vi "Initialize.vi"(8 "error in (no error)":errorcluster, 11 "Configuration":T1) -> (0 "error out":errorcluster, 3 "Configuration Out":T1={"Data Tree Ref"=refnum, "FP Ref"=refnum, "Column Data Type"=[], "Search Clones Up To"=100, "SortOptions"={"Col.pri"=0, "RevDir.pri"=FALSE, "Col.sec"=0, "RevDir.sec"=FALSE}, "Group/Flat (0:group)"=FALSE, "CollapsedNodes"=[], "Show/Hide Cols"=[], "Filtered Paths"=[], "View"=enum."Group By Library", "File Extension Filters"=[], "Filter Global VIs"=FALSE, "Shared"=refnum, "Active Filters"=refnum, "Refresh Rate (ms)"=2000, "App Instance Ring Ref"=refnum, "Processing Q"=refnum, "VI Ref"=refnum})   [LabVIEW 2013, in "LVTM.lvlib"]
uses:
  LVTM.lvlib
  Controls_LVTM/SharedDataDVR.ctl
  Controls_LVTM/View.ctl
  Controls_LVTM/LVTM_Config_Info.ctl
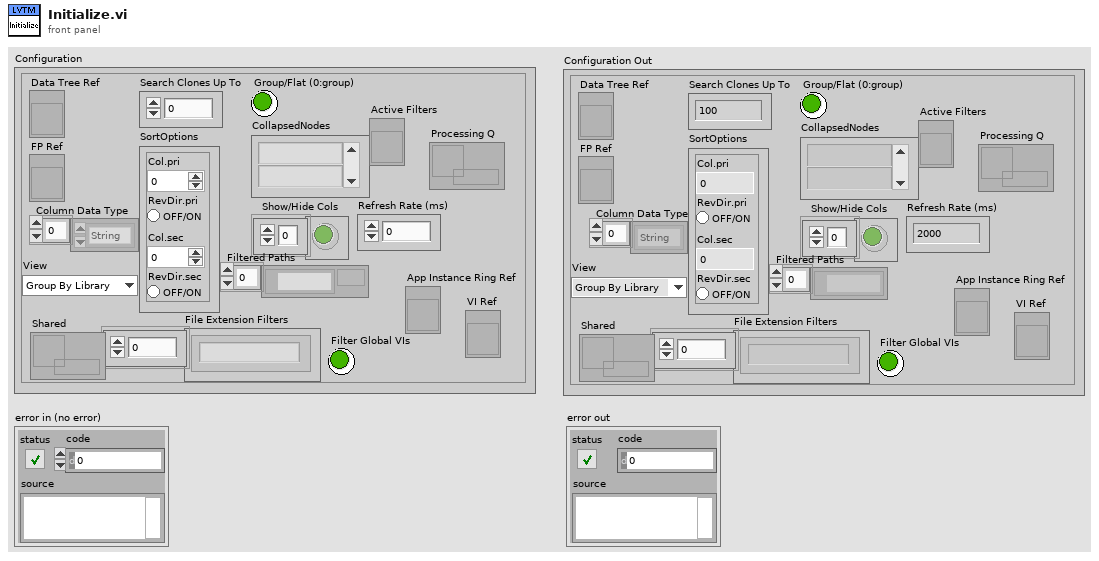
[diagram p1: front panel]
types:
  T1 = typedef "LVTM.lvlib/LVTM_Config_Info.ctl" = cluster{"Data Tree Ref":refnum<vi>, "FP Ref":refnum<vi>, "Column Data Type":enum16{"String", "Numeric"}[], "Search Clones Up To":i32, "SortOptions":cluster{"Col.pri":i32, "RevDir.pri":bool, "Col.sec":i32, "RevDir.sec":bool}, "Group/Flat (0:group)":bool, "CollapsedNodes":string[], "Show/Hide Cols":bool[], "Filtered Paths":path[], "View":T2, "File Extension Filters":string[], "Filter Global VIs":bool, "Shared":refnum<data-value>, "Active Filters":refnum<vi>, "Refresh Rate (ms)":i32, "App Instance Ring Ref":refnum<vi>, "Processing Q":refnum<queue>, "VI Ref":refnum<vi>}
  T2 = typedef "LVTM.lvlib/View.ctl" = enum16{"Group By Library", "Group By Folder", "Flat List"}
  T3 = typedef "LVTM.lvlib/SharedDataDVR.ctl" = cluster{"App":refnum<vi>, "VIs":string[]}
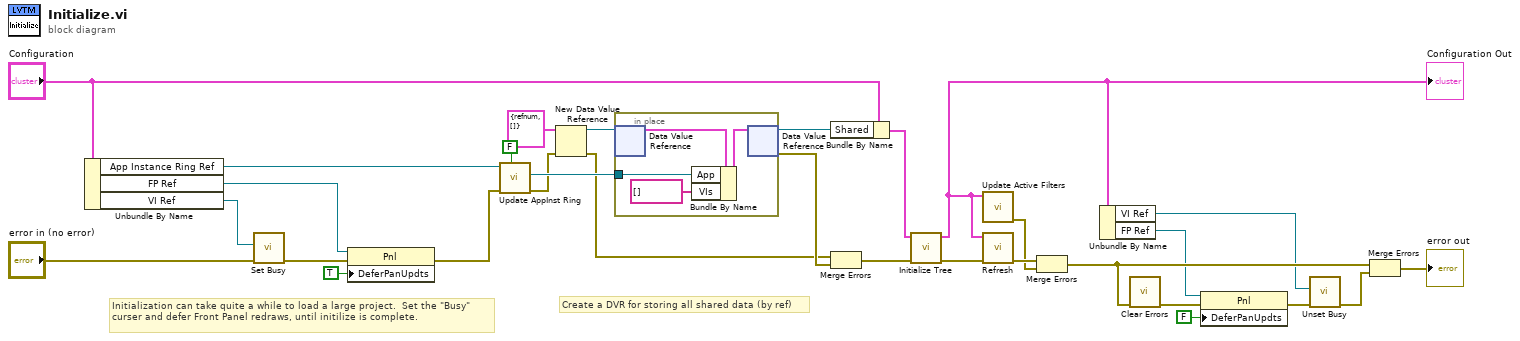
[diagram p0: block diagram]
diagram:
  # "Create a DVR for storing all shared data (by ref)"
  # "Initialization can take quite a while to load a large project.  Set the \"Busy\" curser and defer Front Panel redraws, until initilize is complete."
  n1 = Unbundle By Name("Configuration") -> ("App Instance Ring Ref"=w9:refnum<vi>, "FP Ref"=w14:refnum<vi>, "VI Ref"=w8:refnum<vi>)
  n2 = call <vilib>:"Set Busy.vi"("error in (no error)"="error in (no error)", "VI reference (current VI)"=w8) -> ("error out"=w2:errorcluster)  [unwired: 8 in, 1 out]
  n3 = property class="Pnl"(reference=w14, error in=w2, "DeferPanUpdts"=TRUE ("Defer Panel Updates")) -> (error out=w5:errorcluster)  [unwired: 1 out]
  n4 = call "Update AppInst Ring.vi"("OpenAppDialog"=FALSE ("OK Button"), "error in"=w5, "Ring in"=w9) -> ("error out"=w19:errorcluster, "AppInst out"=w22:refnum<vi>)  [unwired: 6 in, 1 out]
  n5 = New Data Value Reference(data value=T3 {"App"=refnum, "VIs"=[]}, error in=w19) -> (data value reference=w20:refnum<data-value>, error out=w4:errorcluster)
  n6 = in-place {
    in-place-border: w22 -> [w31]
    n7 = in-place-dvr #1(w20) -> (w34:T3)  [unwired: 1 out]
    n8 = Bundle By Name(cluster=w34, "App"=w31, "VIs"=string[] []) -> (w33:T3)
    n9 = in-place-dvr #1(w33) -> (w17:refnum<data-value>, w6:errorcluster)
  }
  n10 = Bundle By Name(cluster="Configuration", "Shared"=w17) -> (w18:T1)
  n11 = Merge Errors(w4, w6) -> (w7:errorcluster)
  n12 = call "Initialize Tree.vi"("error in (no error)"=w7, "Configuration"=w18) -> ("error out"=w29:errorcluster, "Configuration Out"=w16:T1)  [unwired: 8 in]
  "Configuration Out" <- w16
  n13 = call "Update Active Filters.vi"("Configuration"=w16) -> ("error out"=w26:errorcluster)  [unwired: 10 in]
  n14 = call "Refresh.vi"("error in (no error)"=w29, "Configuration"=w16) -> ("error out"=w28:errorcluster)  [unwired: 9 in]
  n15 = Merge Errors(w28, w26) -> (w23:errorcluster)
  n16 = Unbundle By Name(w16) -> ("VI Ref"=w15:refnum<vi>, "FP Ref"=w13:refnum<vi>)
  n17 = call <vilib>:"Clear Errors.vi"("error in (no error)"=w23) -> ("error out"=w24:errorcluster)  [unwired: 5 in, 1 out]
  n18 = property class="Pnl"(reference=w13, error in=w24, "DeferPanUpdts"=FALSE ("Defer Panel Updates")) -> (error out=w25:errorcluster)  [unwired: 1 out]
  n19 = call <vilib>:"Unset Busy.vi"("error in (no error)"=w25, "VI reference (current VI)"=w15) -> ("error out"=w11:errorcluster)  [unwired: 9 in]
  n20 = Merge Errors(w23, w11) -> (→"error out":errorcluster)
